vi "Default Section.vi"(8 "error in (no error)":errorcluster, 11 "Node Ptr":T1 format="%.0x") -> (0 "error out":errorcluster)   [LabVIEW 2019, in "Diagnostics Addon System Explorer.lvlib"]
uses:
  Diagnostics Addon System Explorer.lvlib
  <vilib>/NI VeriStand/Custom Device API/Custom Device API.lvlib
  <vilib>/NI VeriStand/Custom Device Tools/Custom Device Utility Library/Custom Device Utility Library.lvlib
  Shared/SubVIs/Constants.vi
  Shared/Diagnostics Addon Shared.lvlib
  <vilib>/NI VeriStand/Custom Device Tools/Custom Device Utility Library/NI VeriStand - Search for Item by GUID.vi
  <vilib>/NI VeriStand/Custom Device API/Custom Device Item Ref.ctl
panel:
  in  "SHDocVw.IWebBrowser":refnum<k7>(container)
  in  "Settings 6":i64 format="%.0x"
  in  "Settings 5":i64 format="%.0x"
  in  "Settings 4":i64 format="%.0x"
  in  "Settings 3":i64 format="%.0x"
  in  "Settings 2":i64 format="%.0x"
  in  "Settings 1":i64 format="%.0x"
  in  "Header 2":cluster{"Section Name":string}={"Section Name"="Section Default Values"}
  in  "Header":cluster{"Section Name":string}={"Section Name"="Section Item Settings"}
  in  "Description":string
  out "Name":string
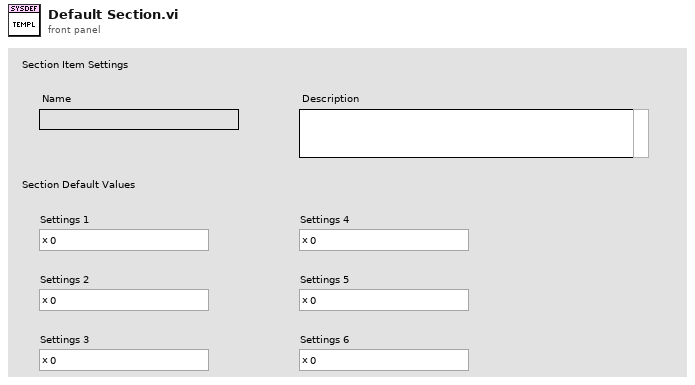
[diagram p1: front panel]
types:
  T1 = typedef "Custom Device API.lvlib/Custom Device Item Ref.ctl" = u64
  T2 = typedef "Custom Device API.lvlib/Custom Device Item Info.ctl" = cluster{"Name":string, "Is Channel":bool, "GUID":string, "Is Waveform":bool}
  T3 = typedef "Custom Device API.lvlib/Custom Device Channel.ctl" = cluster{"Type":T4, "Units":string, "Default Value":dbl, "Faultable":bool, "Scalable":bool}
  T4 = typedef "Custom Device API.lvlib/Custom Device Channel Type.ctl" = enum16{"Input", "Output"}
  T5 = typedef "Custom Device API.lvlib/Custom Device Commands.ctl" = enum16{"Default", "Item renamed", "Shutdown", "Dynamic button pressed"}
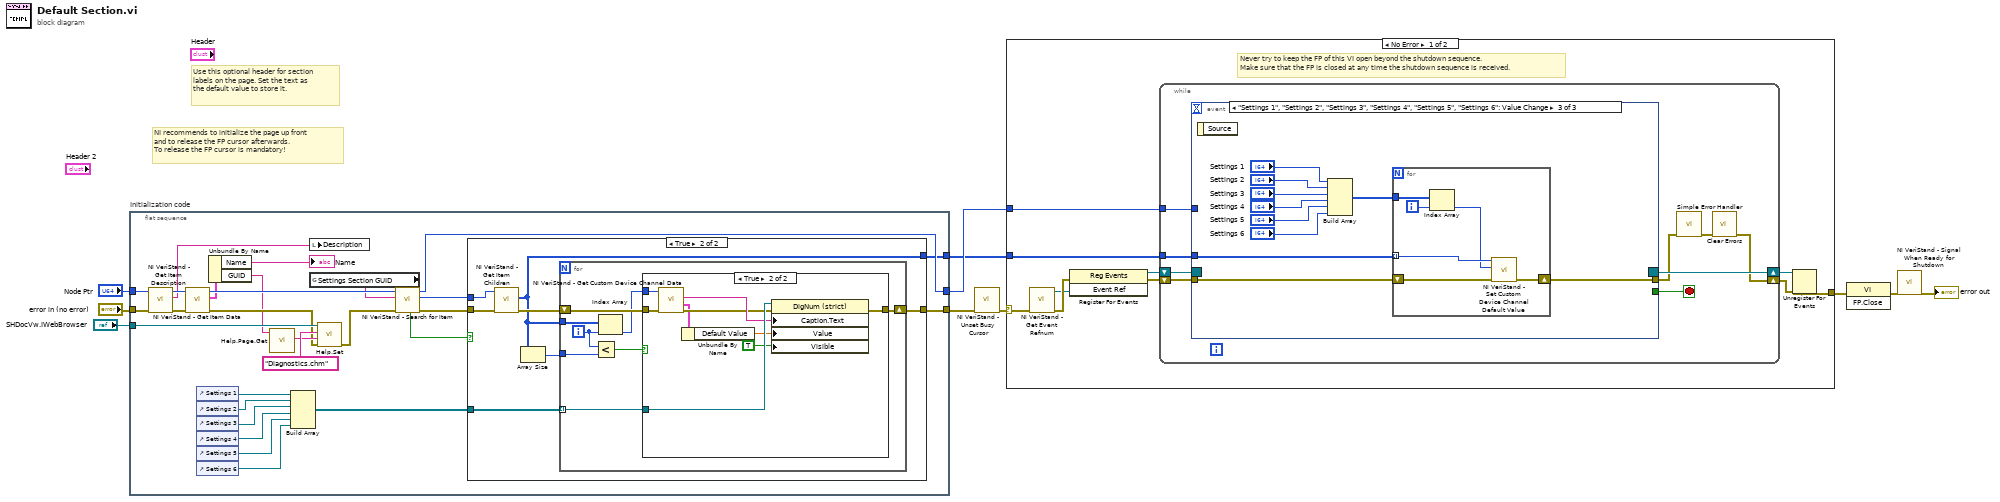
[diagram p0: block diagram]
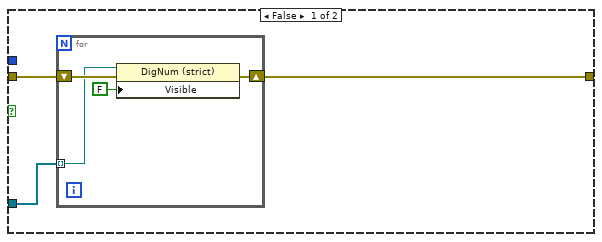
[diagram p2: hidden frame]
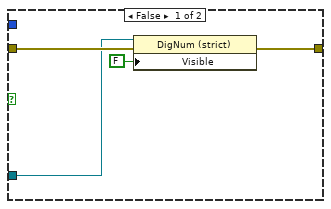
[diagram p3: hidden frame]
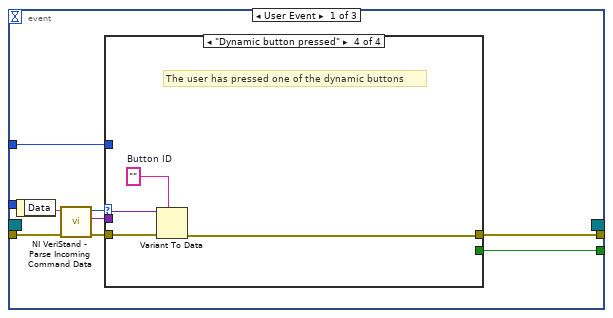
[diagram p4: hidden frame]
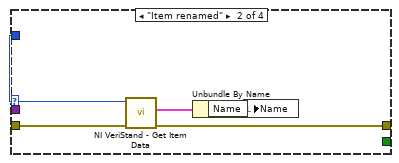
[diagram p6: hidden frame]
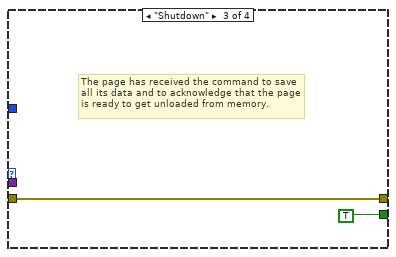
[diagram p7: hidden frame]
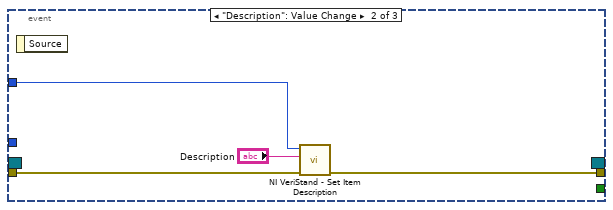
[diagram p8: hidden frame]
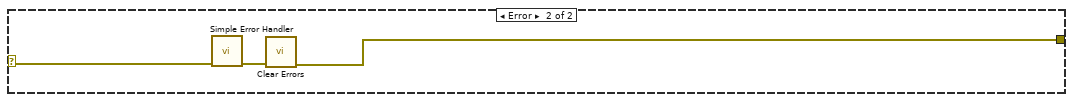
[diagram p9: hidden frame]
diagram:
  # "Use this optional header for section labels on the page. Set the text as the default value to store it."
  # "NI recommends to initialize the page up front\nand to release the FP cursor afterwards.\nTo release the FP cursor is mandatory!"
  n1 = flat-sequence "Initialization code" {
    tunnel: "error in (no error)" -> [w36]
    tunnel: "Node Ptr" -> [w35]
    tunnel: [w20] -> w6
    tunnel: [w19] -> w3
    tunnel: [w17] -> w2
    tunnel: "SHDocVw.IWebBrowser" -> [w14]
    frame #0 {
      n2 = call <vilib>:"NI VeriStand - Get Item Description.vi"("error in (no error)"=w36, "Item Ref in"=w35) -> ("error out"=w33:errorcluster, "Description"=w34:string, "Item Ref out"=w37:T1)  [unwired: 7 out]
      n3 = call <vilib>:"NI VeriStand - Get Item Data.vi"("error in (no error)"=w33, "Item Ref in"=w37) -> ("error out"=w13:errorcluster, "Item Info"=w32:T2, "Item Ref out"=w38:T1)  [unwired: 7 out]
      n4 = control-ref of="Settings 1"() -> (w28:refnum<vi>)
      n5 = control-ref of="Settings 2"() -> (w27:refnum<vi>)
      n6 = control-ref of="Settings 3"() -> (w26:refnum<vi>)
      n7 = control-ref of="Settings 4"() -> (w25:refnum<vi>)
      n8 = control-ref of="Settings 5"() -> (w24:refnum<vi>)
      n9 = control-ref of="Settings 6"() -> (w23:refnum<vi>)
      n10 = Unbundle By Name(w32) -> ("Name"=→"Name":string, "GUID"=w11:string)
      n11 = call "Help.Page.Get.vi"("GUID"=w11) -> ("HTML File"=w15:string)  [unwired: 10 in]
      n12 = Build Array(w28, w27, w26, w25, w24, w23) -> (w22:refnum<vi>[])
      n13 = local write "Description"(w34) -> ()
      n14 = global read "Constants.vi" "Settings Section GUID"() -> (w30:string)
      n15 = call "Help.Set.vi"("error in (no error)"=w13, "HTML File"=w15, "Main CHM File"="Diagnostics.chm", "SHDocVw.IWebBrowser2"=w14) -> ("error out"=w12:errorcluster)  [unwired: 7 in]
      n16 = call-poly <vilib>:"NI VeriStand - Search for Item.vi"("error in"=w12, "Item GUID"=w30, "Section Ref in"=w38) -> ("error out"=w21:errorcluster, "Item Ref"=w18:T1, "Section Ref out"=w19:T1, "Found"=w29:bool)  [unwired: 5 in]
      n17 = case shown="True" w29 {
        tunnel: w22 -> [w41 w52]
        tunnel: w21 -> [w40 w50]
        tunnel: [w39 w51] -> w20
        tunnel: w18 -> [_ w48]
        tunnel: [_ w46] -> w17
        frame False {
          n18 = for {
            tunnel: w41 -> [w44] mode=indexing
            shift-right: [w42] -> w39
            shift-left: w40 -> [w45]
            n19 = property class="DigNum (strict)"(reference=w44, error in=w45, "Visible"=FALSE) -> (error out=w42:errorcluster)  [unwired: 1 out]
          }
        }
        frame True {
          n20 = call <vilib>:"NI VeriStand - Get Item Children.vi"("error in (no error)"=w50, "Item Ref in"=w48) -> ("error out"=w49:errorcluster, "Child Refs"=w46:T1[])  [unwired: 6 in, 2 out]
          n21 = Array Size(array=w46) -> (size(s)=w47:i32)
          n22 = for {
            tunnel: w52 -> [w60] mode=indexing
            shift-right: [w59] -> w51
            shift-left: w49 -> [w57]
            tunnel: w46 -> [w58]
            tunnel: w47 -> [w54]
            i -> [w55]
            n23 = Less?(x=w55, y=w54) -> (x < y?=w53:bool)
            n24 = Index Array(array=w58, index=w55) -> (element=w56:T1)
            n25 = case shown="True" w53 {
              tunnel: w60 -> [w61 w73]
              tunnel: [w62 w72] -> w59
              tunnel: w57 -> [w63 w70]
              tunnel: w56 -> [_ w69]
              frame False {
                n26 = property class="DigNum (strict)"(reference=w61, error in=w63, "Visible"=FALSE) -> (error out=w62:errorcluster)  [unwired: 1 out]
              }
              frame True {
                n27 = call <vilib>:"NI VeriStand - Get Custom Device Channel Data.vi"("error in (no error)"=w70, "Channel Ref in"=w69) -> ("error out"=w67:errorcluster, "Channel"=w66:T3, "Channel Name"=w68:string)  [unwired: 4 in, 3 out]
                n28 = Unbundle By Name(w66) -> ("Default Value"=w65:dbl)
                n29 = property class="DigNum (strict)"(reference=w73, error in=w67, "Caption.Text"=w68, "Value"=w65, "Visible"=TRUE) -> (error out=w72:errorcluster)  [unwired: 1 out]
              }
            }
          }
        }
      }
    }
  }
  n30 = call <vilib>:"NI VeriStand - Unset Busy Cursor.vi"("error in (no error)"=w6) -> ("error out"=w5:errorcluster)  [unwired: 10 out]
  n31 = case shown="No Error" w5 {
    selector: w5 -> [w75 w135]
    tunnel: [w80 w133] -> w10
    tunnel: w3 -> [w76 _]
    tunnel: w2 -> [w74 _]
    frame No Error {
      # "Never try to keep the FP of this VI open beyond the shutdown sequence.\nMake sure that the FP is closed at any time the shutdown sequence is received."
      n32 = call <vilib>:"NI VeriStand - Get Event Refnum.vi"("error in (no error)"=w75) -> ("error out"=w83:errorcluster, "Event Ref"=w79:refnum<user-event>)  [unwired: 9 out]
      n33 = register-events(error in=w83, w79) -> (reference out=w77:refnum<event-registration>, error out=w78:errorcluster)  [unwired: 1 in]
      n34 = while {
        tunnel: w76 -> [w88]
        shift-right: [w85] -> w81
        shift-left: w78 -> [w91]
        shift-right: [w92] -> w82
        shift-left: w77 -> [w90]
        tunnel: w74 -> [w84]
        stop <- w89 stop-if-true
        n35 = event shown="[2] \"Settings 1\", \"Settings 2\", \"Settings 3\", \"Settings 4\", \"Settings 5\", \"Settings 6\": Value Change" {
          selector: w90 -> [_ _ _]
          dyn-events: [_ _ _] -> w92
          timeout: _ -> [_ _ _]
          tunnel: w91 -> [w100 w115 w126]
          tunnel: [w96 _ _] -> w89
          tunnel: [w95 w114 w124] -> w87
          tunnel: w88 -> [w94 w116 _]
          tunnel: w84 -> [_ _ w125]
          event User Event {
            n36 = event-data() -> ("Data"=w99:string)  [unwired: 1 out]
            n37 = call <vilib>:"NI VeriStand - Parse Incoming Command Data.vi"("error in (no error)"=w100, "Incoming data"=w99) -> ("error out"=w98:errorcluster, "Outgoing data"=w93:variant, "Action"=w97:T5)  [unwired: 7 out]
            n38 = case shown="\"Dynamic button pressed\"" w97 {
              tunnel: w98 -> [w101 w106 w107 w112]
              tunnel: [_ _ TRUE _] -> w96
              tunnel: [w101 w103 w107 w109] -> w95
              tunnel: w94 -> [_ w105 _ _]
              tunnel: w93 -> [_ _ _ w111]
              frame "Default", Default {
              }
              frame "Item renamed" {
                n39 = call <vilib>:"NI VeriStand - Get Item Data.vi"("error in (no error)"=w106, "Item Ref in"=w105) -> ("error out"=w103:errorcluster, "Item Info"=w104:T2)  [unwired: 8 out]
                n40 = Unbundle By Name(w104) -> ("Name"=w102:string)
                n41 = local write "Name"(w102) -> ()
              }
              frame "Shutdown" {
                # "The page has received the command to save all its data and to acknowledge that the page is ready to get unloaded from memory."
              }
              frame "Dynamic button pressed" {
                w110 = ""  # Button ID
                # "The user has pressed one of the dynamic buttons"
                n42 = Variant To Data(error in=w112, type=w110, Variant=w111) -> (error out=w109:errorcluster)  [unwired: 1 out]
              }
            }
          }
          event "Description": Value Change {
            n43 = event-data() -> ()  [unwired: 2 out]
            n44 = call <vilib>:"NI VeriStand - Set Item Description.vi"("error in (no error)"=w115, "Description"="Description", "Item Ref in"=w116) -> ("error out"=w114:errorcluster)  [unwired: 8 out]
          }
          event "Settings 1", "Settings 2", "Settings 3", "Settings 4", "Settings 5", "Settings 6": Value Change {
            n45 = event-data() -> ()  [unwired: 2 out]
            n46 = Build Array("Settings 1", "Settings 2", "Settings 3", "Settings 4", "Settings 5", "Settings 6") -> (w117:i64[])
            n47 = for {
              tunnel: w125 -> [w131] mode=indexing
              shift-right: [w130] -> w124
              shift-left: w126 -> [w132]
              tunnel: w117 -> [w129]
              i -> [w127]
              n48 = Index Array(array=w129, index=w127) -> (element=w128:i64)
              n49 = call <vilib>:"NI VeriStand - Set Custom Device Channel Default Value.vi"("error in (no error)"=w132, "Default Value"=w128, "Channel Ref in"=w131) -> ("error out"=w130:errorcluster)  [unwired: 7 in, 1 out]
            }
          }
        }
        n50 = call <vilib>:"Simple Error Handler.vi"("error in (no error)"=w87) -> ("error out"=w86:errorcluster)  [unwired: 1 in, 7 out]
        n51 = call <vilib>:"Clear Errors.vi"("error in (no error)"=w86) -> ("error out"=w85:errorcluster)  [unwired: 1 in, 5 out]
      }
      n52 = Unregister For Events(event registration refnum=w82, error in=w81) -> (error out=w80:errorcluster)
    }
    frame Error {
      n53 = call <vilib>:"Simple Error Handler.vi"("error in (no error)"=w135) -> ("error out"=w134:errorcluster)  [unwired: 1 in, 7 out]
      n54 = call <vilib>:"Clear Errors.vi"("error in (no error)"=w134) -> ("error out"=w133:errorcluster)  [unwired: 1 in, 5 out]
    }
  }
  n55 = invoke class="VI" method="FP.Close"(error in=w10) -> (error out=w9:errorcluster)  [unwired: 2 in, 2 out]
  n56 = call <vilib>:"NI VeriStand - Signal When Ready for Shutdown.vi"("error in (no error)"=w9) -> ("error out"=→"error out":errorcluster)  [unwired: 10 out]
